vi "Shuffle_2D_Array.vi"(10 "Array":sgl[][](array[numeric]), 11 "Byte Stream File in":refnum<file>) -> (2 "sorted 2D array":dbl[][](array[numeric]), 3 "Byte Stream File out":refnum<file>)   [LabVIEW 2020]
uses:
  1807f32a-839a-4780-bb02-3554cfabd9e7.vi
  <vilib>/Array/Sort 2D Array - Pop Stack.vi
  <vilib>/Array/Sort 2D Array - Push Stack.vi
  1807f32a-839a-4780-bb02-3554cfabd9e7.vi/269d4b3b-47f5-49e3-8884-44851e4dd9d5.vi
  1807f32a-839a-4780-bb02-3554cfabd9e7.vi/6d99389c-673d-4efb-bf33-19b32bcf4cf8.vi
panel:
  out "appended array":dbl[](array[numeric])
  out "Array 2":dbl[][](array[numeric])
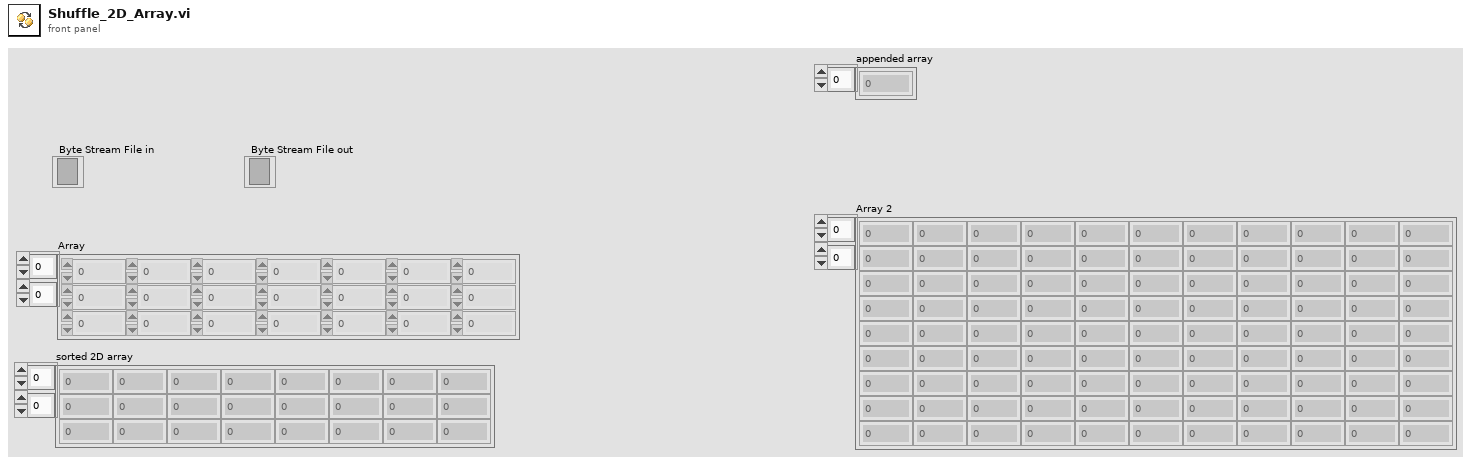
[diagram p1: front panel]
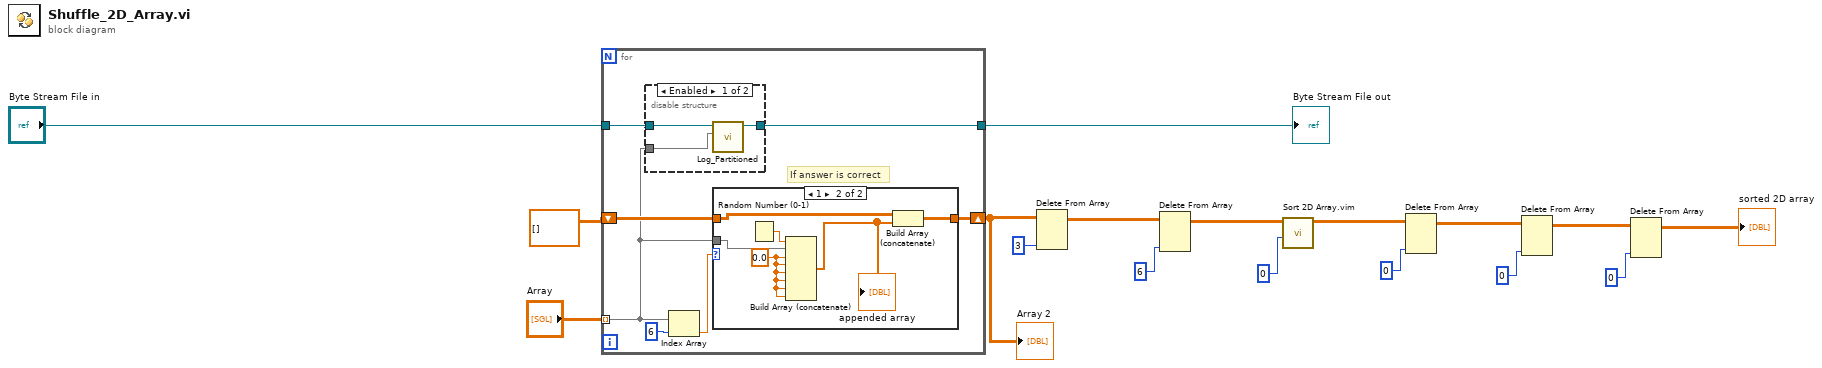
[diagram p0: block diagram]
diagram:
  n1 = for {
    tunnel: "Array" -> [w18] mode=indexing
    shift-right: [w22] -> w12
    shift-left: sgl[][] [] -> [w23]
    tunnel: "Byte Stream File in" -> [w20]
    tunnel: [w19] -> w16
    # "If answer is correct"
    n2 = disable-structure shown="Enabled" {
      disable-tunnel: w20 -> [w27 w28]
      disable-tunnel: [w26 w28] -> w19
      disable-tunnel: w18 -> [w25 _]
      frame Enabled {
        n3 = call "Log_Partitioned.vi"("Array"=w25, "Byte Stream File in"=w27) -> ("Byte Stream File out"=w26:refnum<file>)  [unwired: 9 in]
      }
      frame Disabled {
      }
    }
    n4 = Index Array(array=w18, index=6) -> (element=w21:sgl)
    n5 = case shown="1" w21 {
      tunnel: w18 -> [_ w35]
      tunnel: w23 -> [w29 w33]
      tunnel: [w29 w32] -> w22
      frame Default {
      }
      frame 1 {
        w30 = 0.0
        n6 = Random Number (0-1)() -> (number: 0 to 1=w34:dbl)
        n7 = Build Array (concatenate) "Build Array"(w34, w35, w30, w30, w30, w30, w30, w30) -> (w31:dbl[])
        "appended array" <- w31
        n8 = Build Array (concatenate) "Build Array"(w33, w31) -> (w32:dbl[][])
      }
    }
  }
  "Byte Stream File out" <- w16
  "Array 2" <- w12
  n9 = Delete From Array "Delete From Array"(array=w12, index (col)=3) -> (array with subset deleted=w9:dbl[][])  [unwired: 2 in, 1 out]
  n10 = Delete From Array "Delete From Array"(array=w9, index (col)=6) -> (array with subset deleted=w11:dbl[][])  [unwired: 2 in, 1 out]
  n11 = call "Sort 2D Array.vim"("index"=0, "2D array"=w11) -> ("sorted 2D array"=w14:dbl[][])  [unwired: 8 in, 1 out]
  n12 = Delete From Array "Delete From Array"(array=w14, index (col)=0) -> (array with subset deleted=w5:dbl[][])  [unwired: 2 in, 1 out]
  n13 = Delete From Array "Delete From Array"(array=w5, index (col)=0 ("disabled index (col)")) -> (array with subset deleted=w4:dbl[][])  [unwired: 2 in, 1 out]
  n14 = Delete From Array "Delete From Array"(array=w4, index (col)=0 ("disabled index (col)")) -> (array with subset deleted=→"sorted 2D array":dbl[][])  [unwired: 2 in, 1 out]
